vi "ScanivalveInit.vi"(0 "Scanner IP Address":string, 1 "Sampling Frequency Requested (Hz)":dbl, 2 "Total # of Samples to Collect":i32) -> (3 "TCP Network Connection out":refnum<k5>, 6 "error out":errorcluster)   [LabVIEW 2019]
panel:
  out "Sampling Frequency Set (Hz)":dbl=10.0 format="%#_6f"
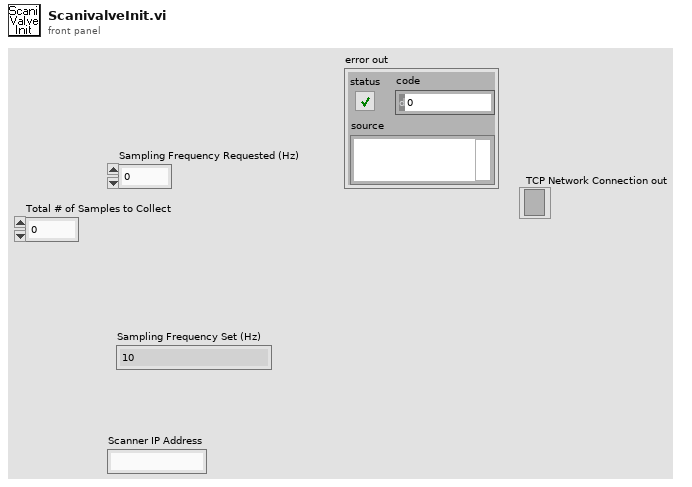
[diagram p1: front panel]
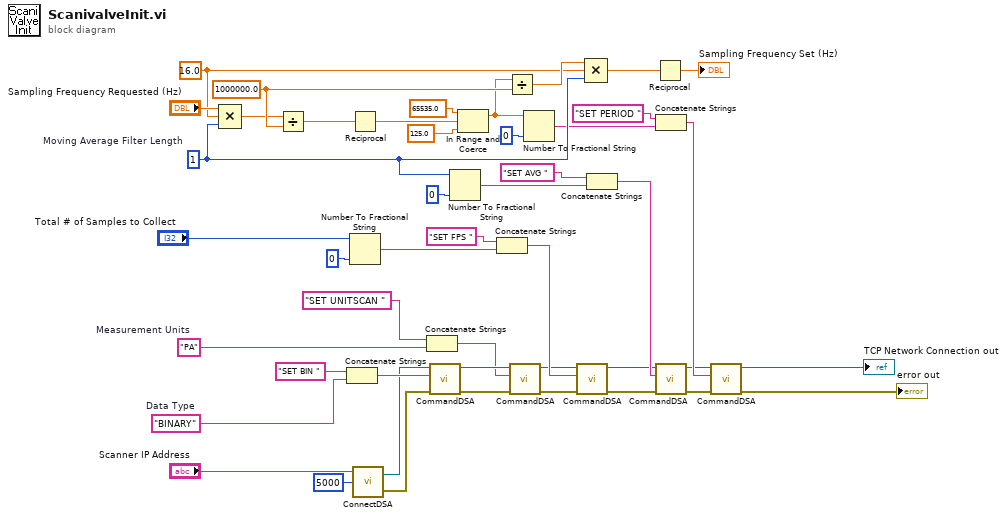
[diagram p0: block diagram]
diagram:
  w38 = i8 1  # Moving Average Filter Length
  w17 = "PA"  # Measurement Units
  w46 = "BINARY"  # Data Type
  w36 = 1000000.0 ("y")
  w32 = 16.0 ("x")
  n1 = Compound Arithmetic op=MULTIPLY("Sampling Frequency Requested (Hz)", w32, w38) -> (w29:dbl)
  n2 = Divide(x=w29, y=w36) -> (x/y=w34:dbl)
  n3 = Concatenate Strings("SET BIN ", w46) -> (w45:string)
  n4 = Reciprocal(x=w34) -> (1/x=w28:dbl)
  n5 = Number To Fractional String(number="Total # of Samples to Collect", precision (6)=i16 0) -> (F-format string=w8:string)  [unwired: 2 in]
  n6 = call "ConnectDSA.vi"("timeout ms (20000)"=5000, "address"="Scanner IP Address") -> ("error out"=w40:errorcluster, "connection ID out"=w42:refnum<k5>)  [unwired: 2 in]
  n7 = Concatenate Strings("SET UNITSCAN ", w17) -> (w16:string)
  n8 = call "CommandDSA.vi"("error in (no error)"=w40, "command"=w45, "connection ID"=w42) -> ("error out"=w41:errorcluster, "connection ID out"=w43:refnum<k5>)  [unwired: 1 in, 2 out]
  n9 = Number To Fractional String(number=w38, precision (6)=i16 0) -> (F-format string=w20:string)  [unwired: 2 in]
  n10 = In Range and Coerce(upper limit=65535.0, x=w28, lower limit=125.0) -> (coerced(x)=w33:dbl)  [unwired: 1 out]
  n11 = Concatenate Strings("SET FPS ", w8) -> (w10:string)
  n12 = Divide(x=w33, y=w36) -> (x/y=w35:dbl)
  n13 = call "CommandDSA.vi"("error in (no error)"=w41, "command"=w16, "connection ID"=w43) -> ("error out"=w3:errorcluster, "connection ID out"=w2:refnum<k5>)  [unwired: 1 in, 2 out]
  n14 = Number To Fractional String(number=w33, precision (6)=i16 0) -> (F-format string=w24:string)  [unwired: 2 in]
  n15 = call "CommandDSA.vi"("error in (no error)"=w3, "command"=w10, "connection ID"=w2) -> ("error out"=w4:errorcluster, "connection ID out"=w5:refnum<k5>)  [unwired: 1 in, 2 out]
  n16 = Compound Arithmetic op=MULTIPLY(w35, w32, w38) -> (w31:dbl)
  n17 = Concatenate Strings("SET AVG ", w20) -> (w22:string)
  n18 = Reciprocal(x=w31) -> (1/x=→"Sampling Frequency Set (Hz)":dbl)
  n19 = Concatenate Strings("SET PERIOD ", w24) -> (w39:string)
  n20 = call "CommandDSA.vi"("error in (no error)"=w4, "command"=w22, "connection ID"=w5) -> ("error out"=w15:errorcluster, "connection ID out"=w14:refnum<k5>)  [unwired: 1 in, 2 out]
  n21 = call "CommandDSA.vi"("error in (no error)"=w15, "command"=w39, "connection ID"=w14) -> ("error out"=→"error out":errorcluster, "connection ID out"=→"TCP Network Connection out":refnum<k5>)  [unwired: 1 in, 2 out]
